vi "move_to_index.vi"(4 "error in (no error)":errorcluster, 6 "Request data":variant, 7 "Python session in":refnum<k35>) -> (0 "error out":errorcluster, 2 "Response data":variant, 3 "Python session out":refnum<k35>)   [LabVIEW 2022 SP3]
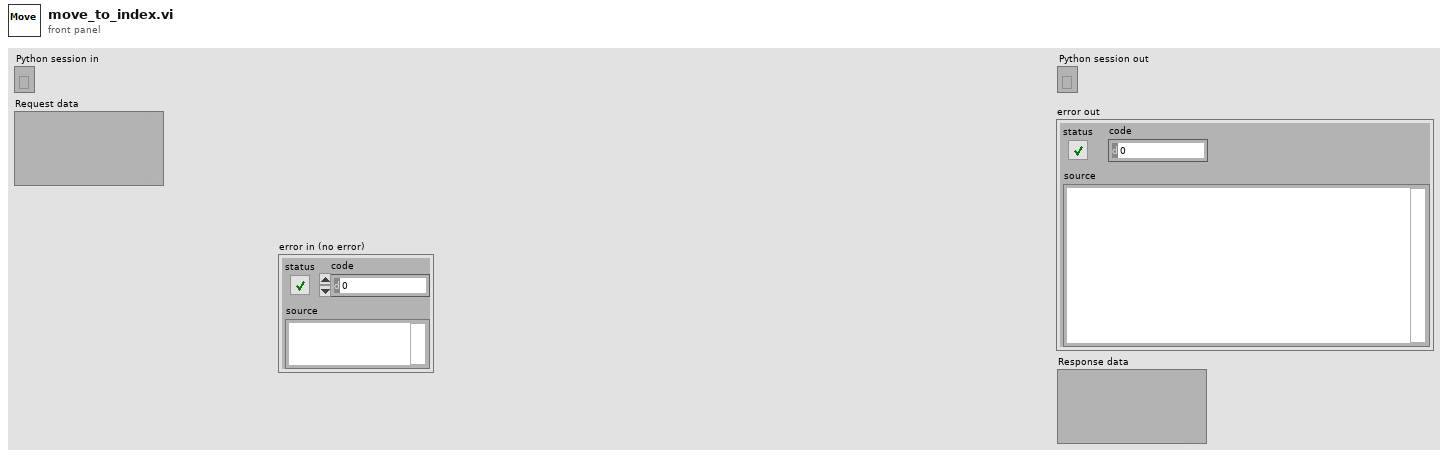
[diagram p1: front panel]
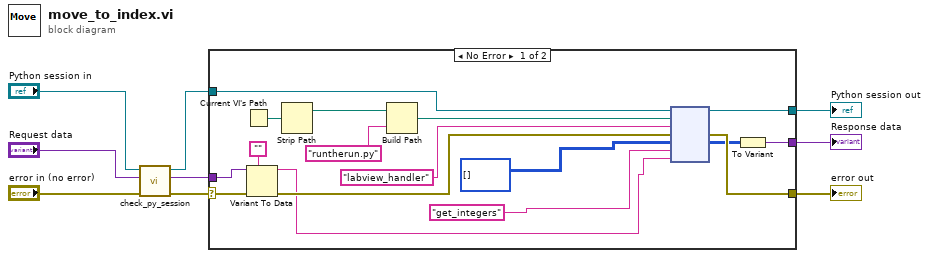
[diagram p0: block diagram]
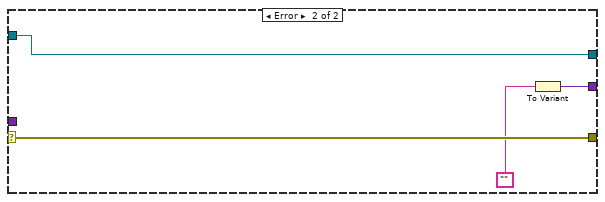
[diagram p2: hidden frame]
diagram:
  n1 = call "check_py_session.vi"("error in"="error in (no error)", "Request data"="Request data", "Python session in"="Python session in") -> ("error out"=w3:errorcluster, "Response data"=w4:variant, "Python session out"=w5:refnum<k35>)  [unwired: 2 in]
  n2 = case shown="No Error" w3 {
    selector: w3 -> [w17 w30]
    tunnel: w5 -> [w26 w29]
    tunnel: [w20 w29] -> w9
    tunnel: w4 -> [w18 _]
    tunnel: [w15 w30] -> w2
    tunnel: [w13 w27] -> w1
    frame No Error {
      n3 = Current VI's Path() -> (path=w22:path)
      n4 = Variant To Data(error in=w17, type="", Variant=w18) -> (data=w11:string, error out=w16:errorcluster)
      n5 = Strip Path(path=w22) -> (stripped path=w21:path)  [unwired: 1 out]
      n6 = Build Path(base path=w21, name or relative path="runtherun.py") -> (appended path=w24:path)
      n7 = node(w26, w24, "labview_handler" ("function name"), w16, i32[][] [], "get_integers", w11) -> (w20:refnum<k35>, w15:errorcluster, w14:i32[][])  [unwired: 2 in, 2 out]
      n8 = To Variant(anything=w14) -> (Variant=w13:variant)
    }
    frame Error {
      n9 = To Variant(anything="") -> (Variant=w27:variant)
    }
  }
  "error out" <- w2
  "Python session out" <- w9
  "Response data" <- w1
